vi "Get Qualified Name.vi"(8 "error in (no error)":errorcluster {"code" format="Error %.0f"}, 11 "Interface Documenation In":refnum<class "Interface Documenation.lvclass">) -> (0 "error out":errorcluster {"code" format="Error %.0f"}, 2 "Qualified Name":string, 3 "Interface Documenation Out":refnum<class "Interface Documenation.lvclass">)   [LabVIEW 2023, in "VIDoc Parsing.lvlib" / "Interface Documenation.lvclass"]
uses:
  Interface Documenation.lvclass
  Interface Documenation.lvclass/Interface Documenation.ctl
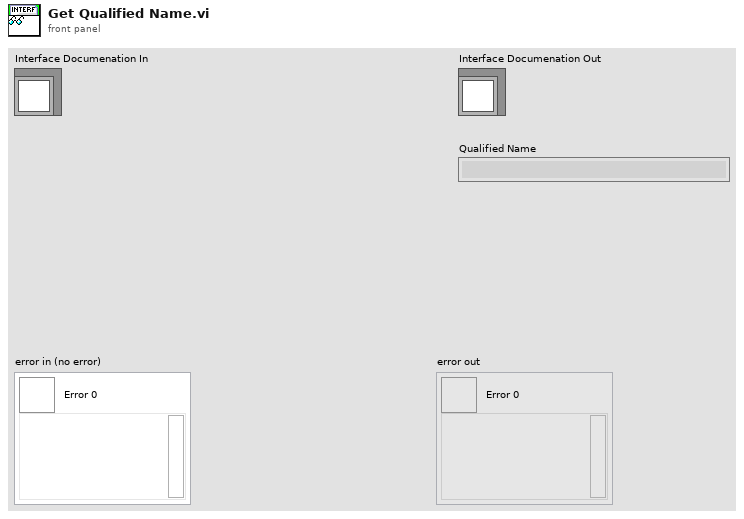
[diagram p1: front panel]
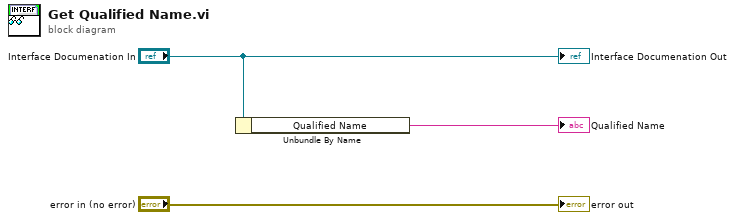
[diagram p0: block diagram]
diagram:
  n1 = Unbundle By Name("Interface Documenation In") -> ("Qualified Name"=→"Qualified Name":string)
  "error out" <- "error in (no error)"
  "Interface Documenation Out" <- "Interface Documenation In"
